vi "Check Library Tag.vi"(8 "error in":errorcluster, 11 "Library Icon Data in":refnum<class "Library Icon Data.lvclass">) -> (0 "error out":errorcluster, 3 "Library Icon Data out":refnum<class "Library Icon Data.lvclass">)   [LabVIEW 2020, in "Library Icon Data.lvclass"]
doc: "Reads the tag in the XML of the library to verify the proper tag name was used for the save version of the library."
uses:
  Library Icon Data.lvclass
  Library Icon Data.lvclass/Library Icon Data.ctl
  e7d835d4-484a-418e-bbba-5da4f525552a.vi
  <vilib>/xml/NI_XML.lvlib
  <vilib>/xml/Load XML File.vi
  <resource>/objmgr/DOMUserDefRef.rc
  <vilib>/xml/Close Reference(Node).vi
  <vilib>/xml/XPath/Get First Matched Node (String).vi
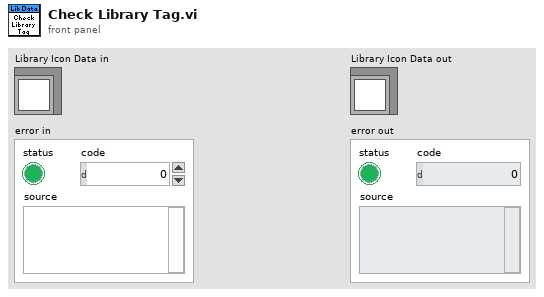
[diagram p1: front panel]
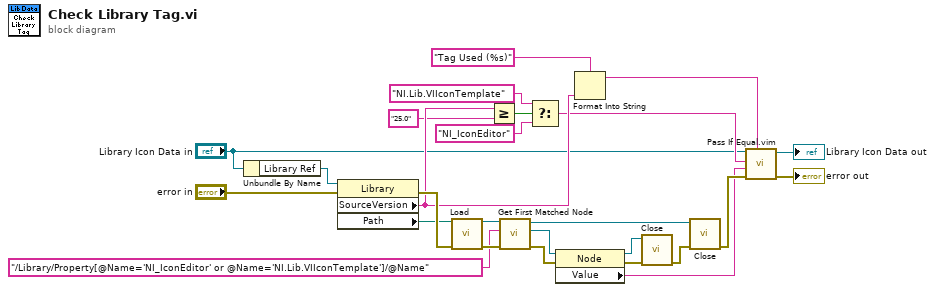
[diagram p0: block diagram]
diagram:
  n1 = Unbundle By Name("Library Icon Data in") -> ("Library Ref"=w17:refnum<vi>)
  n2 = property class="Library"(reference=w17, error in="error in") -> (error out=w24:errorcluster, "SourceVersion"=w5:string, "Path"=w11:path)  [unwired: 1 out]
  n3 = call-poly <vilib>:"Load.vi"("path to XML document"=w11, "error in (no error)"=w24) -> ("DOM document out"=w9:refnum<k20>, "error out"=w20:errorcluster)  [unwired: 11 in, 1 out]
  n4 = Greater Or Equal?(x=w5, y="25.0") -> (x >= y?=w16:bool)
  n5 = call-poly <vilib>:"Get First Matched Node.vi"("error in (no error)"=w20, "XPath expression"="/Library/Property[@Name='NI_IconEditor' or @Name='NI.Lib.VIIconTemplate']/@Name", "node in"=w9) -> ("error out"=w23:errorcluster, "node result"=w12:refnum<k20>, "node out"=w8:refnum<k20>)  [unwired: 6 in]
  n6 = Select(t="NI.Lib.VIIconTemplate", s=w16, f="NI_IconEditor") -> (s? t:f=w4:string)
  n7 = property class="Node"(reference=w12, error in=w23) -> (reference out=w10:refnum<k20>, error out=w21:errorcluster, "Value"=w7:string)
  n8 = Format Into String(format string="Tag Used (%s)" ("Description"), w5) -> (resulting string=w3:string)  [unwired: 2 in, 1 out]
  n9 = call-poly <vilib>:"Close.vi"("error in (no error)"=w21, "node"=w10) -> ("error out"=w22:errorcluster)  [unwired: 7 in]
  n10 = call-poly <vilib>:"Close.vi"("error in (no error)"=w22, "node"=w8) -> ("error out"=w19:errorcluster)  [unwired: 7 in]
  n11 = call "Pass If Equal.vim"("Description"=w3, "error in (no error)"=w19, "Actual"=w7, "Expected"=w4, "LUnit Test Case In"="Library Icon Data in") -> ("error out"=→"error out":errorcluster, "LUnit Test Case Out"=→"Library Icon Data out":refnum<class "Library Icon Data.lvclass">)  [unwired: 5 in]
